vi "Date.vi"(1 "DeviceName":string, 2 "Format Date/Time String":string) -> (0 "fileName":string)   [LabVIEW 2019]
panel:
  out "First Part of name":string
  out "Last Part of name":string
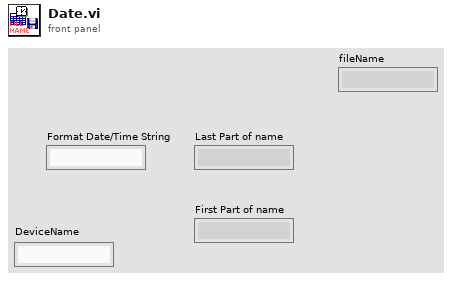
[diagram p1: front panel]
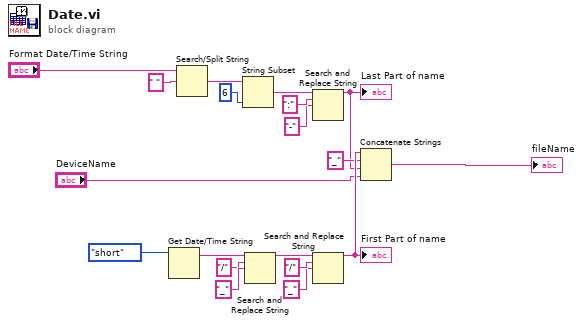
[diagram p0: block diagram]
diagram:
  n1 = Get Date/Time String(date format (0)=enum16{"short", "long", "abbreviated"}."short") -> (date string=w8:string)  [unwired: 2 in, 1 out]
  n2 = Search/Split String(string="Format Date/Time String", search string/char (-)=" ") -> (match + rest of string=w17:string)  [unwired: 1 in, 2 out]
  n3 = String Subset(string=w17, length (rest)=6 ("length (rest)")) -> (substring=w15:string)  [unwired: 1 in]
  n4 = Search and Replace String(input string=w8, search string="/", replace string="_" ("replace string (\"\")")) -> (result string=w11:string)  [unwired: 5 in, 3 out]
  n5 = Search and Replace String(input string=w15, search string=":", replace string="-" ("replace string (\"\")")) -> (result string=w3:string)  [unwired: 5 in, 3 out]
  "Last Part of name" <- w3
  n6 = Search and Replace String(input string=w11, search string="/", replace string="_" ("replace string (\"\")")) -> (result string=w5:string)  [unwired: 5 in, 3 out]
  "First Part of name" <- w5
  n7 = Concatenate Strings(w5, "_" ("string"), w3, "DeviceName") -> (→"fileName":string)
